vi "ProjFile_Read File.vi"(8 "error in":errorcluster, 11 "file (use dialog)":path) -> (0 "error out":errorcluster, 1 "Resource Data":T1, 2 "Project Data":T4, 3 "LangData File Path":path, 5 "Assumed Project Path":path)   [LabVIEW 2013, in "SET Project Data.lvlib"]
doc: "ProjFile_Read File.vi\n\nOpen a SET Project File. Returns Project Data and Resource Data."
uses:
  SET Project Data.lvlib
  Types/ProjFile_Project Data.ctl
  Types/ProjFile_Menu Data.ctl
  Types/ProjFile_VI Data.ctl
  Types/ProjFile_GObject Data.ctl
  Types/ProjFile_Resources Data.ctl
  Types/ProjFile_Language Entry.ctl
  Types/ProjFile_Resource Entry.ctl
panel:
  out "Project Name":string
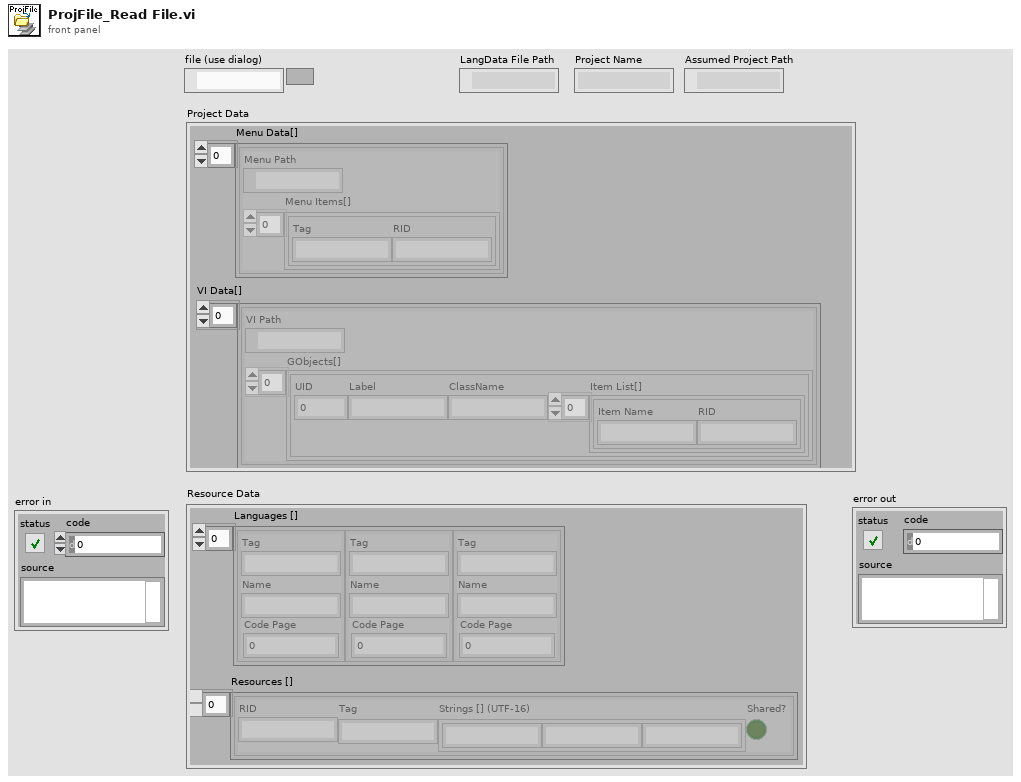
[diagram p1: front panel]
types:
  T1 = typedef "SET Project Data.lvlib/ProjFile_Resources Data.ctl" = cluster{"Languages []":T2[], "Resources []":T3[]}
  T2 = typedef "SET Project Data.lvlib/ProjFile_Language Entry.ctl" = cluster{"Tag":string, "Name":string, "Code Page":u16}
  T3 = typedef "SET Project Data.lvlib/ProjFile_Resource Entry.ctl" = cluster{"RID":string, "Tag":string, "Strings [] (UTF-16)":string[], "Shared?":bool}
  T4 = typedef "SET Project Data.lvlib/ProjFile_Project Data.ctl" = cluster{"Menu Data[]":T5[], "VI Data[]":T6[]}
  T5 = typedef "SET Project Data.lvlib/ProjFile_Menu Data.ctl" = cluster{"Menu Path":path, "Menu Items[]":cluster{"Tag":string, "RID":string}[]}
  T6 = typedef "SET Project Data.lvlib/ProjFile_VI Data.ctl" = cluster{"VI Path":path, "GObjects[]":T7[]}
  T7 = typedef "SET Project Data.lvlib/ProjFile_GObject Data.ctl" = cluster{"UID":i32, "Label":string, "ClassName":string, "Item List[]":cluster{"Item Name":string, "RID":string}[]}
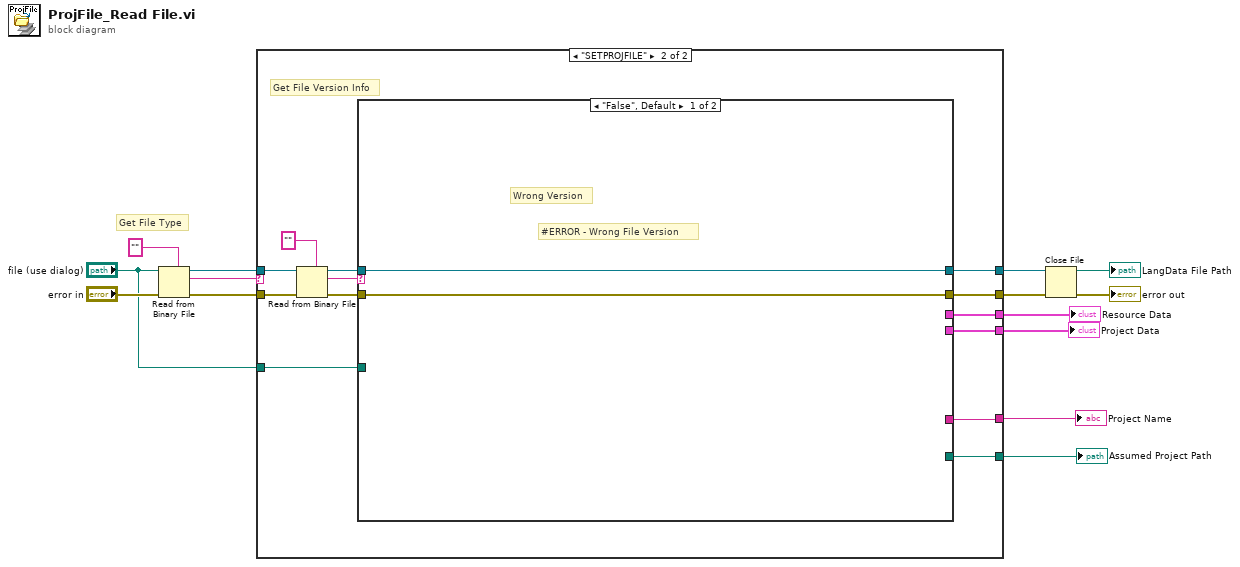
[diagram p0: block diagram]
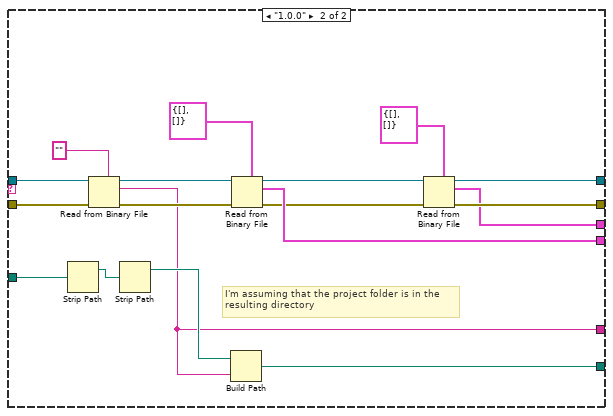
[diagram p3: hidden frame]
diagram:
  # "Get File Type"
  n1 = Read from Binary File(5:"", 8:"error in", 11:"file (use dialog)") -> (0:w11:errorcluster, 2:w13:string, 3:w12:refnum<file>)  [unwired: 3 in, 1 out]
  n2 = case shown="\"SETPROJFILE\"" w13 {
    tunnel: w12 -> [w16 w29]
    tunnel: w11 -> [w15 w28]
    tunnel: [w16 w23] -> w10
    tunnel: [w15 w22] -> w9
    tunnel: [_ w21] -> w4
    tunnel: [_ w20] -> w5
    tunnel: "file (use dialog)" -> [_ w19]
    tunnel: [_ w18] -> w2
    tunnel: [_ w17] -> w1
    frame "False", Default {
      # "#ERROR - Wrong File Type"
    }
    frame "SETPROJFILE" {
      # "Get File Version Info"
      n3 = Read from Binary File(5:"" ("data type"), 8:w28, 11:w29) -> (0:w24:errorcluster, 2:w26:string, 3:w25:refnum<file>)  [unwired: 3 in, 1 out]
      n4 = case shown="\"False\", Default" w26 {
        tunnel: w25 -> [w31 w49]
        tunnel: w24 -> [w30 w48]
        tunnel: [w31 w34] -> w23
        tunnel: [w30 w35] -> w22
        tunnel: [_ w40] -> w21
        tunnel: [_ w38] -> w20
        tunnel: w19 -> [_ w43]
        tunnel: [_ w39] -> w18
        tunnel: [_ w32] -> w17
        frame "False", Default {
          # "#ERROR - Wrong File Version"
          # "Wrong Version"
        }
        frame "1.0.0" {
          # "I'm assuming that the project folder is in the\nresulting directory"
          n5 = Strip Path(path=w43) -> (stripped path=w42:path)  [unwired: 1 out]
          n6 = Read from Binary File(5:"" ("data type"), 8:w48, 11:w49) -> (0:w45:errorcluster, 2:w40:string, 3:w46:refnum<file>)  [unwired: 3 in, 1 out]
          n7 = Strip Path(path=w42) -> (stripped path=w41:path)  [unwired: 1 out]
          n8 = Build Path(base path=w41, name or relative path=w40) -> (appended path=w39:path)
          n9 = Read from Binary File(5:T4 {"Menu Data[]"=[], "VI Data[]"=[]}, 8:w45, 11:w46) -> (0:w36:errorcluster, 2:w38:T4, 3:w37:refnum<file>)  [unwired: 3 in, 1 out]
          n10 = Read from Binary File(5:T1 {"Languages []"=[], "Resources []"=[]} ("Resource Data"), 8:w36, 11:w37) -> (0:w35:errorcluster, 2:w32:T1, 3:w34:refnum<file>)  [unwired: 3 in, 1 out]
        }
      }
    }
  }
  "Project Data" <- w5
  "Project Name" <- w4
  "Assumed Project Path" <- w2
  "Resource Data" <- w1
  n11 = Close File(refnum=w10, error in=w9) -> (path=→"LangData File Path":path, error out=→"error out":errorcluster)
